vi "save_image_subtraction_value_to_textfile.vi"(10 "Image subtraction\nvalue":i32) -> ()   [LabVIEW 2011]
uses:
  Action-Init-Update-Get.ctl
  <vilib>/Utility/file.llb/Write To Spreadsheet File (I64).vi
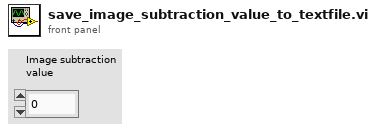
[diagram p1: front panel]
types:
  T1 = typedef "Action-Init-Update-Get.ctl" = enum16{"Initialize", "Update", "Get"}
  T2 = cluster{"Path":string, "Filestem":string, "Filestem incl time t":string, "Date":string}
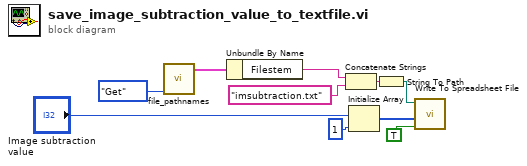
[diagram p0: block diagram]
diagram:
  n1 = call "file_pathnames.vi"("Action"=Action-Init-Update-Get."Get") -> ("File-path\n-names"=w6:T2)  [unwired: 10 in]
  n2 = Unbundle By Name(w6) -> ("Filestem"=w5:string)
  n3 = Concatenate Strings(w5, "imsubtraction.txt" ("new file path (Not A Path if cancelled)")) -> (w7:string)
  n4 = Initialize Array("Image subtraction\nvalue", 1 ("Dimension")) -> (w3:i32[])
  n5 = String To Path(string=w7) -> (path=w9:path)
  n6 = call-poly <vilib>:"Write To Spreadsheet File.vi"("append to file? (new file:F)"=TRUE, "1D data"=w3, "file path (dialog if empty)"=w9) -> ()  [unwired: 5 in, 1 out]
